vi "main.vi"() -> ()   [LabVIEW 2023]
doc: "The main VI file. \n\nThis file contains the logic and elements. \n\nInput values are united in cluster which as type def. defined. \nEnum is type def as well.\n\nThe calculation is in a loop."
uses:
  Controls/inputTypeDef.ctl
  Controls/enumTypeDef.ctl
panel:
  out "Output":dbl
  in  "?":bool
  in  "Input Values":T1
  # "Calculator"
  # "="
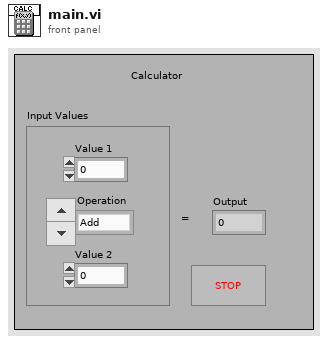
[diagram p1: front panel]
types:
  T1 = typedef "inputTypeDef.ctl" = cluster{"Operation":T2, "Value 1":dbl, "Value 2":dbl}
  T2 = typedef "enumTypeDef.ctl" = enum16{"Add", "Subtract", "Multiply", "Divide"}
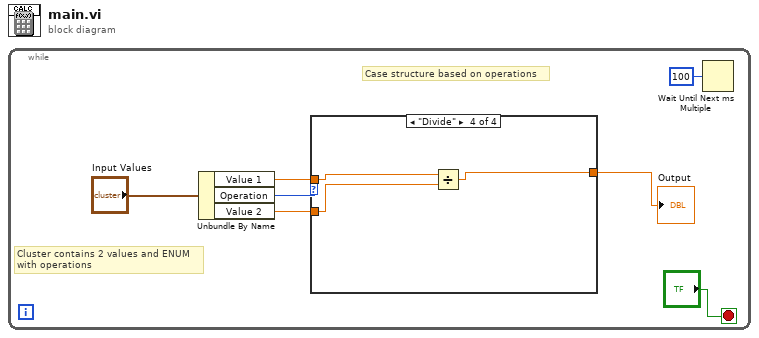
[diagram p0: block diagram]
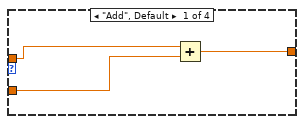
[diagram p2: hidden frame]
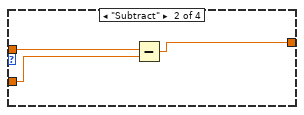
[diagram p3: hidden frame]
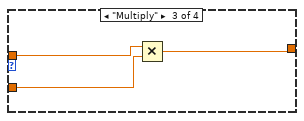
[diagram p4: hidden frame]
diagram:
  n1 = while {
    stop <- "?" stop-if-true
    # "Case structure based on operations"
    # "Cluster contains 2 values and ENUM\nwith operations"
    n2 = Unbundle By Name("Input Values") -> ("Value 1"=w3:dbl, "Operation"=w4:T2, "Value 2"=w2:dbl)
    n3 = case shown="\"Divide\"" w4 {
      tunnel: w3 -> [w10 w13 w16 w19]
      tunnel: w2 -> [w9 w12 w15 w18]
      tunnel: [w8 w11 w14 w17] -> w1
      frame "Add", Default {
        n4 = Add(x=w10, y=w9) -> (x+y=w8:dbl)
      }
      frame "Subtract" {
        n5 = Subtract(x=w13, y=w12) -> (x-y=w11:dbl)
      }
      frame "Multiply" {
        n6 = Multiply(x=w16, y=w15) -> (x*y=w14:dbl)
      }
      frame "Divide" {
        n7 = Divide(x=w19, y=w18) -> (x/y=w17:dbl)
      }
    }
    "Output" <- w1
    n8 = Wait Until Next ms Multiple(millisecond multiple=u32 100) -> ()  [unwired: 1 out]
  }
